vi "dvp Vi Set Rgb Gain.vi"(7 "bGain":sgl, 9 "gGain":sgl, 10 "rGain":sgl, 11 "handle":u32) -> (3 "function return":u32(ring))   [LabVIEW 2018, in "LabViewDVPCamera.lvlib"]
doc: "LabviewDvp2Api dvpStatus dvpViSetRgbGain(dvpHandle handle, float rGain, float gGain, float bGain);"
uses:
  LabViewDVPCamera.lvlib
  LabViewDVPCamera/LabViewDVPCamera.dll
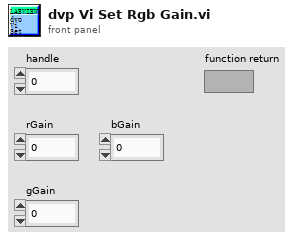
[diagram p1: front panel]
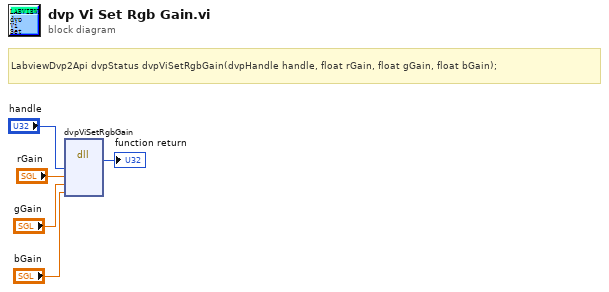
[diagram p0: block diagram]
diagram:
  # "LabviewDvp2Api dvpStatus dvpViSetRgbGain(dvpHandle handle, float rGain, float gGain, float bGain);"
  n1 = dll-call lib="C:/Program Files (x86)/DVP2 Labview cn 64/Sample/LabViewDVPCamera/LabViewDVPCamera.*" fn="dvpViSetRgbGain"("handle"="handle", "rGain"="rGain", "gGain"="gGain", "bGain"="bGain") -> (→"function return":u32)  [unwired: 7 in, 2 out]
